vi "Write Routing Number.vi"(8 "error in (no error)":errorcluster, 10 "Routing Number":string, 11 "AChecking in":refnum<class "AChecking.lvclass">) -> (0 "error out":errorcluster, 3 "AChecking out":refnum<class "AChecking.lvclass">)   [LabVIEW 2020, in "AChecking.lvclass"]
uses:
  AChecking.lvclass
  AChecking.lvclass/AChecking.ctl
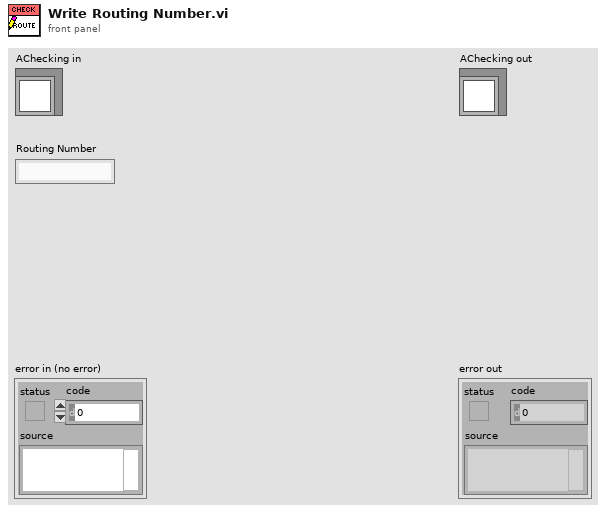
[diagram p1: front panel]
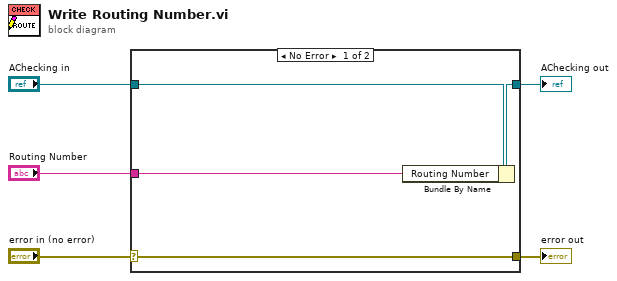
[diagram p0: block diagram]
diagram:
  n1 = case shown="No Error" "error in (no error)" {
    selector: "error in (no error)" -> [w9 w10]
    tunnel: [w9 w10] -> w4
    tunnel: [w7 w11] -> w2
    tunnel: "AChecking in" -> [w8 w11]
    tunnel: "Routing Number" -> [w6 _]
    frame No Error {
      n2 = Bundle By Name(cluster=w8, "Routing Number"=w6) -> (w7:refnum<class "AChecking.lvclass">)
    }
    frame Error {
    }
  }
  "error out" <- w4
  "AChecking out" <- w2
